vi "slider stepper action stack.vi"(7 "stack action":T2, 8 "action list IN":T1[](array[typedef]), 9 "slider setter action":T1=enum."void", 11 "command stack In":T1[](array[typedef])) -> (1 "slider setter action OUT":T1=enum."void", 2 "stack is empty ?":bool, 3 "command stack OUT":T1[](array[typedef]))   [LabVIEW 2018]
uses:
  stack action -- control.ctl
  slider setter action.ctl
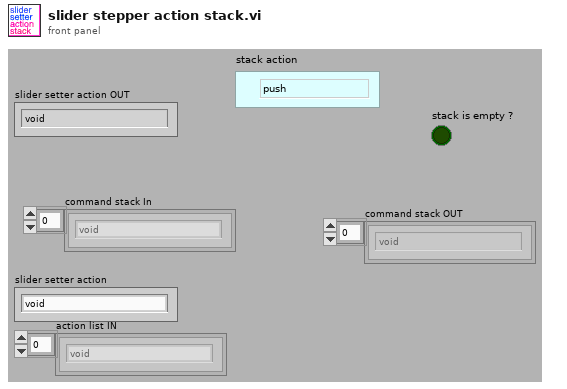
[diagram p1: front panel]
types:
  T1 = typedef "slider setter action.ctl" = enum16{"--update circle", "set slider moves", "cursor moves", "current pos changed", "init", "void"}
  T2 = typedef "stack action -- control.ctl" = enum16{"push", "pop", "check", "init"}
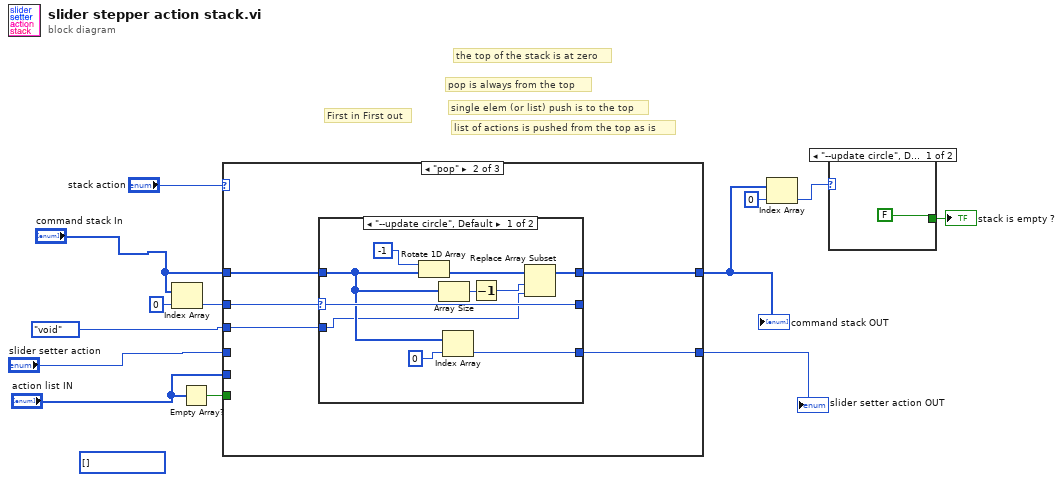
[diagram p0: block diagram]
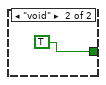
[diagram p2: hidden frame]
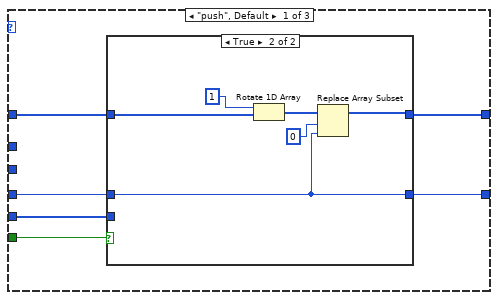
[diagram p3: hidden frame]
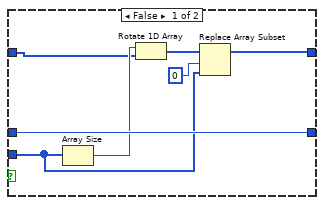
[diagram p4: hidden frame]
diagram:
  (unwired) T1[] [] items=["--update circle", "set slider moves", "cursor moves", "current pos changed", "init", "void"]
  # "list of actions is pushed from the top as is"
  # "single elem (or list) push is to the top"
  # "pop is always from the top"
  # "First in First out"
  # "the top of the stack is at zero"
  n1 = Index Array(array="command stack In", index=0) -> (element=w10:T1)
  n2 = Empty Array?(array="action list IN") -> (empty?=w12:bool)
  n3 = case shown="\"pop\"" "stack action" {
    tunnel: [w19 w37 w51] -> w3
    tunnel: "command stack In" -> [w18 w36 w51]
    tunnel: w10 -> [_ w35 _]
    tunnel: [w14 w34 w52] -> w1
    tunnel: "slider setter action" -> [w17 _ w52]
    tunnel: w12 -> [w16 _ _]
    tunnel: "action list IN" -> [w15 _ _]
    tunnel: slider_setter_action."void" ("slider setter action") -> [_ w33 _]
    frame "push", Default {
      n4 = case shown="True" w16 {
        tunnel: [w20 w27] -> w19
        tunnel: w18 -> [w24 w29]
        tunnel: w17 -> [w26 w30]
        tunnel: w15 -> [w21 _]
        tunnel: [w26 w30] -> w14
        frame False {
          n5 = Array Size(array=w21) -> (size(s)=w25:i32)
          n6 = Rotate 1D Array(1:w24, 2:w25) -> (0:w23:T1[])
          n7 = Replace Array Subset(array=w23, new element=w21, index=0) -> (w20:T1[])
        }
        frame True {
          n8 = Rotate 1D Array(1:w29, 2:1) -> (0:w32:T1[])
          n9 = Replace Array Subset(array=w32, new element=w30, index=0) -> (w27:T1[])
        }
      }
    }
    frame "pop" {
      n10 = case shown="\"--update circle\", Default" w35 {
        selector: w35 -> [w45 w49]
        tunnel: [w41 w50] -> w37
        tunnel: w36 -> [w42 w50]
        tunnel: [w46 w48] -> w34
        tunnel: [w45 w49] -> _
        tunnel: w33 -> [w38 w48]
        frame "--update circle", Default {
          n11 = Rotate 1D Array(1:w42, 2:-1) -> (0:w40:T1[])
          n12 = Array Size(array=w42) -> (size(s)=w43:i32)
          n13 = Index Array(array=w42, index=0) -> (element=w46:T1)
          n14 = Decrement(x=w43) -> (x-1=w39:i32)
          n15 = Replace Array Subset(array=w40, new element=w38, index=w39) -> (w41:T1[])
        }
        frame "void" {
        }
      }
    }
    frame "check" {
    }
  }
  "command stack OUT" <- w3
  "slider setter action OUT" <- w1
  n16 = Index Array(array=w3, index=0) -> (element=w8:T1)
  n17 = case shown="\"--update circle\", Default" w8 {
    tunnel: [FALSE TRUE] -> w7
    frame "--update circle", Default {
    }
    frame "void" {
    }
  }
  "stack is empty ?" <- w7
